vi "BuiltProcedureInfo.vi"(0 "Parameter Data Type String":string, 1 "Length":i16, 2 "Parameter Data Type":i16, 3 "Parameter I/O Type":u8, 4 "Parameter Name":string) -> (5 "Info":string)   [LabVIEW 2011]
doc: "Construit l'information relative aux entrée/ssorties de la requête"
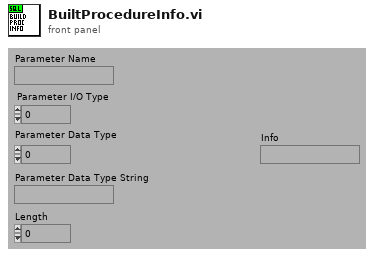
[diagram p1: front panel]
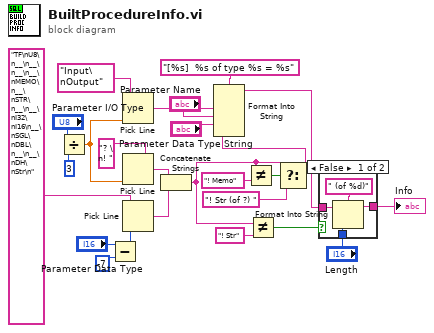
[diagram p0: block diagram]
diagram:
  n1 = Divide(x="Parameter I/O Type", y=u8 3) -> (x/y=w12:dbl)
  n2 = Subtract(x="Parameter Data Type", y=i16 -7) -> (x-y=w15:i16)
  n3 = Pick Line(multi-line string="Input\nOutput", line index=w12) -> (output string=w19:string)  [unwired: 1 out]
  n4 = Pick Line(multi-line string="? \n! ", line index=w12) -> (output string=w11:string)  [unwired: 1 out]
  n5 = Pick Line(multi-line string="TF\nU8\n__\n__\n__\n__\nMEMO\n__\nSTR\n__\n__\nI32\nI16\n__\nSGL\nDBL\n__\n__\nDH\nStr\n", line index=w15) -> (output string=w1:string)  [unwired: 1 out]
  n6 = Concatenate Strings(w11, w1) -> (w2:string)
  n7 = Not Equal?(x=w2, y="! Memo") -> (x != y?=w8:bool)
  n8 = Not Equal?(x=w2, y="! Str" ("f")) -> (x != y?=w24:bool)
  n9 = Select(t=w2, s=w8, f="! Str (of ?) ") -> (s? t:f=w7:string)
  n10 = Format Into String(format string="[%s]  %s of type %s = %s", "Parameter Name", w19, "Parameter Data Type String", w7) -> (resulting string=w10:string)  [unwired: 2 in, 1 out]
  n11 = case shown="False" w24 {
    tunnel: [w28 w30] -> w23
    tunnel: w10 -> [w27 w30]
    tunnel: "Length" -> [w26 _]
    frame False {
      n12 = Format Into String(format string=" (of %d)", initial string=w27, w26) -> (resulting string=w28:string)  [unwired: 1 in, 1 out]
    }
    frame True {
    }
  }
  "Info" <- w23
